vi "Lookup Services of Type.vi"(7 "Type":refnum<class>, 8 "error in (no error)":errorcluster, 11 "Vecto in":refnum<class "Vecto.lvclass">) -> (0 "error out":errorcluster, 2 "Services":refnum<class "Service.lvclass">[](array[class]), 3 "Vecto out":refnum<class "Vecto.lvclass">)   [LabVIEW 2020, in "Vecto.lvlib" / "Vecto.lvclass"]
uses:
  Vecto.lvclass
  Service/Service.lvclass
  Vecto.lvclass/Vecto.ctl
  Service Container/Service Container.lvclass
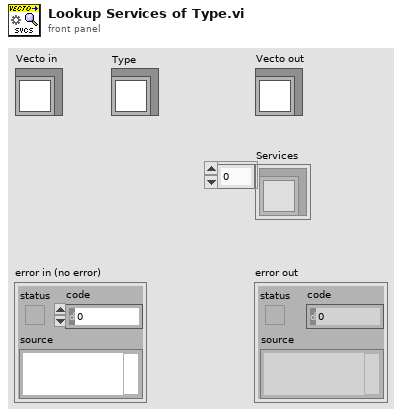
[diagram p1: front panel]
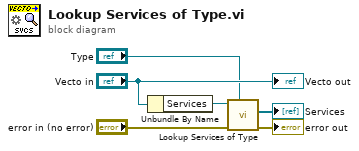
[diagram p0: block diagram]
diagram:
  n1 = Unbundle By Name("Vecto in") -> ("Services"=w5:refnum<class "Service Container.lvclass">)
  n2 = call "Lookup Services of Type.vi"("Type"="Type", "error in (no error)"="error in (no error)", "Service Container in"=w5) -> ("error out"=→"error out":errorcluster, "Services"=→"Services":refnum<class "Service.lvclass">[])  [unwired: 6 in, 1 out]
  "Vecto out" <- "Vecto in"
